vi "Copy Value.vi"(10 "From":refnum<class "Type.lvclass">, 11 "Entity in":refnum<class "Entity.lvclass">) -> (2 "error out":errorcluster, 3 "Entity out":refnum<class "Entity.lvclass">)   [LabVIEW 2020, in "Conditu2.lvlib" / "Columns.lvlib" / "Entity.lvclass"]
uses:
  Entity.lvclass
  Type/Type.lvclass
  Entity.lvclass/Entity.ctl
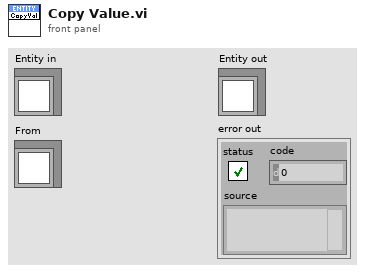
[diagram p1: front panel]
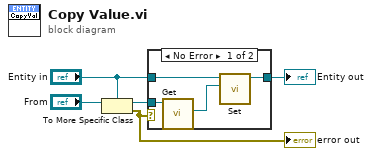
[diagram p0: block diagram]
diagram:
  n1 = To More Specific Class(target class="Entity in", reference="From") -> (specific class reference=w5:refnum<class "Entity.lvclass">, error out=w2:errorcluster)  [unwired: 1 in]
  "error out" <- w2
  n2 = case shown="No Error" w2 {
    tunnel: w5 -> [w9 _]
    tunnel: "Entity in" -> [w7 w10]
    tunnel: [w6 w10] -> w1
    frame No Error {
      n3 = call "Get.vi"("Entity in"=w9) -> ("Value"=w8:refnum<class "Entity.lvclass">)  [unwired: 10 in]
      n4 = call "Set.vi"("Value"=w8, "Entity in"=w7) -> ("Entity out"=w6:refnum<class "Entity.lvclass">)  [unwired: 9 in]
    }
    frame Error {
    }
  }
  "Entity out" <- w1
